vi "trajectory_sinewave.vi"(9 "amplitude":dbl, 10 "counter input":dbl format="%#_13g", 11 "frequency":dbl) -> (2 "sine wave":dbl(graph), 3 "counter output":dbl)   [LabVIEW 2021]
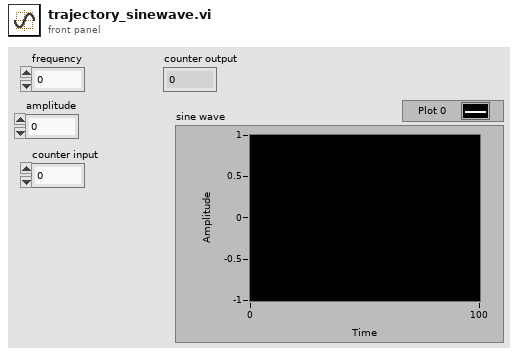
[diagram p1: front panel]
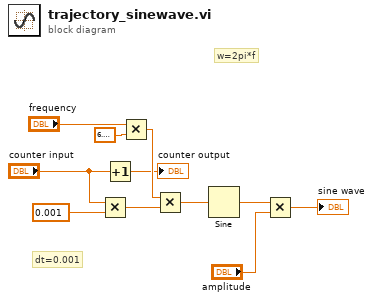
[diagram p0: block diagram]
diagram:
  # "w=2pi*f"
  # "dt=0.001"
  n1 = Multiply(x="counter input", y=0.001) -> (x*y=w7:dbl)
  n2 = Increment(x="counter input") -> (x+1=→"counter output":dbl)
  n3 = Multiply(x="frequency", y=6.283185307179586) -> (x*y=w9:dbl)
  n4 = Multiply(x=w9, y=w7) -> (x*y=w5:dbl)
  n5 = Sine(x=w5) -> (sin(x)=w8:dbl)
  n6 = Multiply(x=w8, y="amplitude") -> (x*y=→"sine wave":dbl)
